vi "hora min seg.vi"(11 "Total time in seconds":dbl) -> (1 "Sec":dbl, 2 "Min":dbl, 3 "H":dbl)   [LabVIEW 2018]
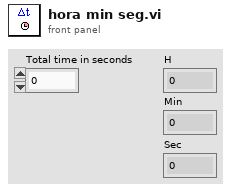
[diagram p1: front panel]
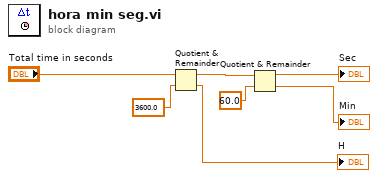
[diagram p0: block diagram]
diagram:
  n1 = Quotient & Remainder(x="Total time in seconds", y=3600.0) -> (x-y*floor(x/y)=w4:dbl, floor(x/y)=→"H":dbl)
  n2 = Quotient & Remainder(x=w4, y=60.0) -> (x-y*floor(x/y)=→"Sec":dbl, floor(x/y)=→"Min":dbl)
